vi "Read Digital Input.vi"(7 "Unit Address (1)":i16=1, 8 "error in (no error)":errorcluster {"code" format="%.0x"}, 10 "Digital Input (1)":i16=1, 11 "VISA resource name":refnum<visa-resource-name>) -> (0 "error out":errorcluster {"code" format="%.0x"}, 2 "Digital Input Value":bool, 3 "VISA resource name out":refnum<visa-resource-name>)   [LabVIEW 2010]
doc: "This VI is used to read Digital Input values."
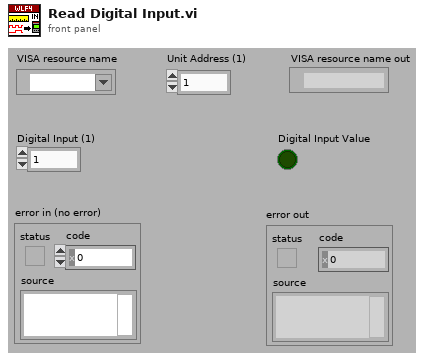
[diagram p1: front panel]
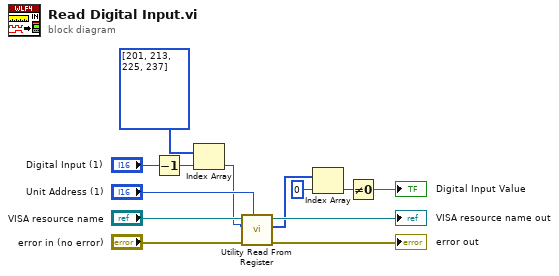
[diagram p0: block diagram]
diagram:
  n1 = Decrement(x="Digital Input (1)") -> (x-1=w5:i16)
  n2 = Index Array(array=i32[] [201, 213, 225, 237], index=w5) -> (element=w2:i32)
  n3 = call "Utility Read From Register.vi"("Unit Address (1)"="Unit Address (1)", "error in (no error)"="error in (no error)", "Register Address (0)"=w2, "VISA resource name"="VISA resource name") -> ("error out"=→"error out":errorcluster, "Data"=w8:i16[], "VISA resource name out"=→"VISA resource name out":refnum<visa-resource-name>)  [unwired: 5 in]
  n4 = Index Array(array=w8, index=0) -> (element=w7:i16)
  n5 = Not Equal To 0?(x=w7) -> (x != 0?=→"Digital Input Value":bool)
